vi "故障分解.vi"(3 "名称":string[](array[string]), 5 "故障输入口":string[](array[string])) -> (0 "故障等级":dbl, 1 "输出数组":string[][](array[string]), 2 "故障显示":string[][](array[string]))   [LabVIEW 2013]
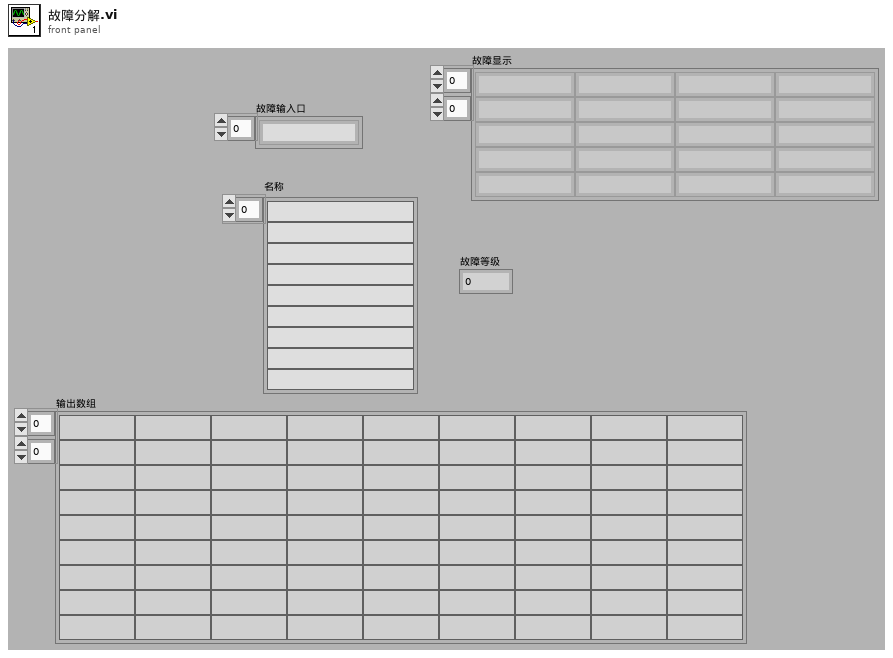
[diagram p1: front panel]
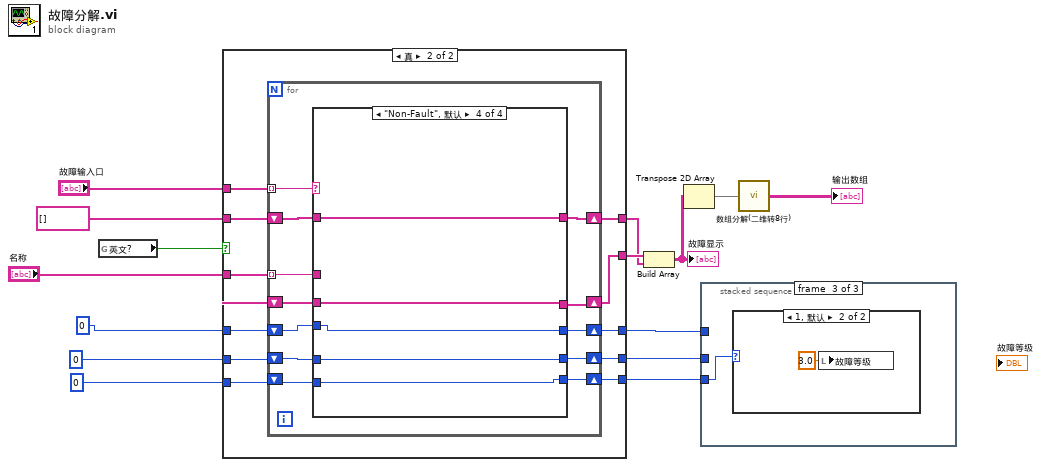
[diagram p0: block diagram]
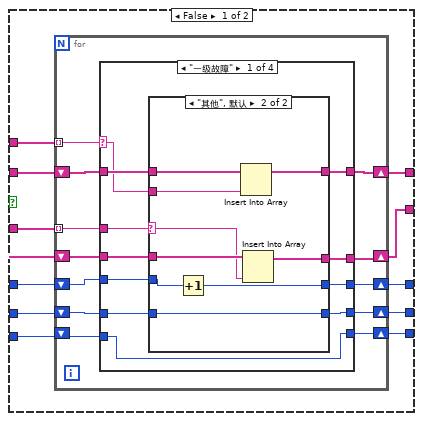
[diagram p2: hidden frame]
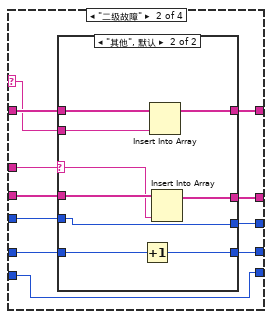
[diagram p4: hidden frame]
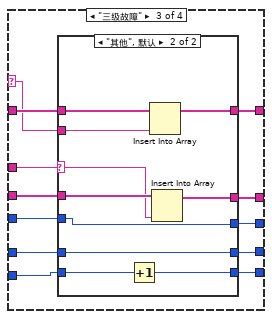
[diagram p6: hidden frame]
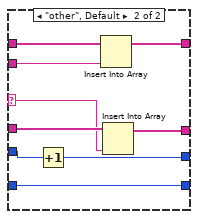
[diagram p10: hidden frame]
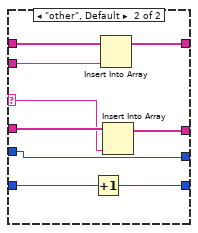
[diagram p12: hidden frame]
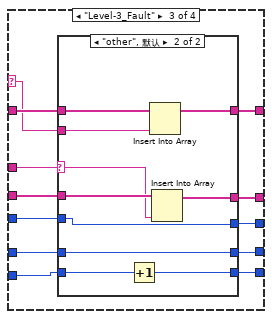
[diagram p13: hidden frame]
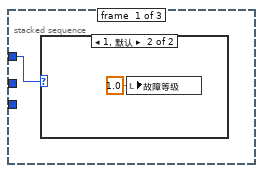
[diagram p15: hidden frame]
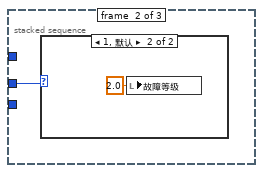
[diagram p17: hidden frame]
diagram:
  n1 = global read "中英文全局-8.6.vi" "英文?"() -> (w1:bool)
  n2 = case shown="真" w1 {
    tunnel: "名称" -> [w26 w129]
    tunnel: string[] [] -> [w25 w128]
    tunnel: 0 ("数值") -> [w24 w127]
    tunnel: 0 ("数值") -> [w23 w126]
    tunnel: 0 ("数值") -> [w22 w125]
    tunnel: [w21 w124] -> w9
    tunnel: [w20 w123] -> w8
    tunnel: [w19 w122] -> w7
    tunnel: [w18 w121] -> w6
    tunnel: [w17 w120] -> w5
    tunnel: "故障输入口" -> [w16 w119]
    frame False {
      n3 = for {
        tunnel: w16 -> [w38] mode=indexing
        tunnel: w26 -> [w35] mode=indexing
        shift-right: [w37] -> w20
        shift-left: w25 -> [w36]
        shift-right: [w33] -> w21
        shift-left: w25 -> [w34]
        shift-right: [w31] -> w19
        shift-left: w24 -> [w32]
        shift-right: [w29] -> w18
        shift-left: w23 -> [w30]
        shift-right: [w27] -> w17
        shift-left: w22 -> [w28]
        n4 = case shown="\"一级故障\"" w38 {
          selector: w38 -> [w47 w71 w96 _]
          tunnel: [w49 w73 w98 w118] -> w37
          tunnel: w36 -> [w48 w72 w97 w118]
          tunnel: w35 -> [w46 w70 w95 _]
          tunnel: w34 -> [w45 w69 w94 w117]
          tunnel: [w44 w68 w93 w117] -> w33
          tunnel: w32 -> [w43 w67 w92 w116]
          tunnel: [w42 w66 w91 w116] -> w31
          tunnel: w30 -> [w40 w65 w90 w115]
          tunnel: [w41 w64 w89 w115] -> w29
          tunnel: w28 -> [w39 w63 w88 w114]
          tunnel: [w39 w63 w87 w114] -> w27
          frame "一级故障" {
            n5 = case shown="\"其他\", 默认" w46 {
              selector: w46 -> [_ w57]
              tunnel: [w53 w62] -> w49
              tunnel: w48 -> [w53 w61]
              tunnel: w47 -> [_ w60]
              tunnel: w45 -> [w52 w59]
              tunnel: [w52 w58] -> w44
              tunnel: [w51 w55] -> w42
              tunnel: w43 -> [w51 w56]
              tunnel: [w50 w54] -> w41
              tunnel: w40 -> [w50 w54]
              frame "保留" {
              }
              frame "其他", Default {
                n6 = Increment(x=w56) -> (x+1=w55:i32)
                n7 = Insert Into Array(array=w61, new element=w60) -> (w62:string[])  [unwired: 1 in]
                n8 = Insert Into Array(array=w59, new element=w57) -> (w58:string[])  [unwired: 1 in]
              }
            }
          }
          frame "二级故障" {
            n9 = case shown="\"其他\", 默认" w70 {
              selector: w70 -> [_ w81]
              tunnel: [w77 w86] -> w73
              tunnel: w72 -> [w77 w85]
              tunnel: w71 -> [_ w84]
              tunnel: w69 -> [w76 w83]
              tunnel: [w76 w82] -> w68
              tunnel: [w75 w80] -> w66
              tunnel: w67 -> [w75 w80]
              tunnel: w65 -> [w74 w79]
              tunnel: [w74 w78] -> w64
              frame "保留" {
              }
              frame "其他", Default {
                n10 = Increment(x=w79) -> (x+1=w78:i32)
                n11 = Insert Into Array(array=w85, new element=w84) -> (w86:string[])  [unwired: 1 in]
                n12 = Insert Into Array(array=w83, new element=w81) -> (w82:string[])  [unwired: 1 in]
              }
            }
          }
          frame "三级故障" {
            n13 = case shown="\"其他\", 默认" w95 {
              selector: w95 -> [_ w108]
              tunnel: [w103 w113] -> w98
              tunnel: w97 -> [w103 w112]
              tunnel: w96 -> [_ w111]
              tunnel: w94 -> [w102 w110]
              tunnel: [w102 w109] -> w93
              tunnel: [w101 w107] -> w91
              tunnel: w92 -> [w101 w107]
              tunnel: w90 -> [w100 w106]
              tunnel: [w100 w106] -> w89
              tunnel: w88 -> [w99 w105]
              tunnel: [w99 w104] -> w87
              frame "保留" {
              }
              frame "其他", Default {
                n14 = Increment(x=w105) -> (x+1=w104:i32)
                n15 = Insert Into Array(array=w112, new element=w111) -> (w113:string[])  [unwired: 1 in]
                n16 = Insert Into Array(array=w110, new element=w108) -> (w109:string[])  [unwired: 1 in]
              }
            }
          }
          frame "无故障", Default {
          }
        }
      }
    }
    frame True {
      n17 = for {
        tunnel: w119 -> [w141] mode=indexing
        tunnel: w129 -> [w138] mode=indexing
        shift-right: [w140] -> w123
        shift-left: w128 -> [w139]
        shift-right: [w136] -> w124
        shift-left: w128 -> [w137]
        shift-right: [w134] -> w122
        shift-left: w127 -> [w135]
        shift-right: [w132] -> w121
        shift-left: w126 -> [w133]
        shift-right: [w130] -> w120
        shift-left: w125 -> [w131]
        n18 = case shown="\"Non-Fault\", 默认" w141 {
          selector: w141 -> [w150 w174 w199 _]
          tunnel: [w152 w176 w201 w221] -> w140
          tunnel: w139 -> [w151 w175 w200 w221]
          tunnel: w138 -> [w149 w173 w198 _]
          tunnel: w137 -> [w148 w172 w197 w220]
          tunnel: [w147 w171 w196 w220] -> w136
          tunnel: w135 -> [w146 w170 w195 w219]
          tunnel: [w145 w169 w194 w219] -> w134
          tunnel: w133 -> [w143 w168 w193 w218]
          tunnel: [w144 w167 w192 w218] -> w132
          tunnel: w131 -> [w142 w166 w191 w217]
          tunnel: [w142 w166 w190 w217] -> w130
          frame "Level-1_Fault" {
            n19 = case shown="\"rsv\"" w149 {
              selector: w149 -> [_ w160]
              tunnel: [w156 w165] -> w152
              tunnel: w151 -> [w156 w164]
              tunnel: w150 -> [_ w163]
              tunnel: w148 -> [w155 w162]
              tunnel: [w155 w161] -> w147
              tunnel: [w154 w158] -> w145
              tunnel: w146 -> [w154 w159]
              tunnel: [w153 w157] -> w144
              tunnel: w143 -> [w153 w157]
              frame "rsv" {
              }
              frame "other", Default {
                n20 = Increment(x=w159) -> (x+1=w158:i32)
                n21 = Insert Into Array(array=w164, new element=w163) -> (w165:string[])  [unwired: 1 in]
                n22 = Insert Into Array(array=w162, new element=w160) -> (w161:string[])  [unwired: 1 in]
              }
            }
          }
          frame "Level-2_Fault" {
            n23 = case shown="\"rsv\"" w173 {
              selector: w173 -> [_ w184]
              tunnel: [w180 w189] -> w176
              tunnel: w175 -> [w180 w188]
              tunnel: w174 -> [_ w187]
              tunnel: w172 -> [w179 w186]
              tunnel: [w179 w185] -> w171
              tunnel: [w178 w183] -> w169
              tunnel: w170 -> [w178 w183]
              tunnel: w168 -> [w177 w182]
              tunnel: [w177 w181] -> w167
              frame "rsv" {
              }
              frame "other", Default {
                n24 = Increment(x=w182) -> (x+1=w181:i32)
                n25 = Insert Into Array(array=w188, new element=w187) -> (w189:string[])  [unwired: 1 in]
                n26 = Insert Into Array(array=w186, new element=w184) -> (w185:string[])  [unwired: 1 in]
              }
            }
          }
          frame "Level-3_Fault" {
            n27 = case shown="\"other\", 默认" w198 {
              selector: w198 -> [_ w211]
              tunnel: [w206 w216] -> w201
              tunnel: w200 -> [w206 w215]
              tunnel: w199 -> [_ w214]
              tunnel: w197 -> [w205 w213]
              tunnel: [w205 w212] -> w196
              tunnel: [w204 w210] -> w194
              tunnel: w195 -> [w204 w210]
              tunnel: w193 -> [w203 w209]
              tunnel: [w203 w209] -> w192
              tunnel: w191 -> [w202 w208]
              tunnel: [w202 w207] -> w190
              frame "rsv" {
              }
              frame "other", Default {
                n28 = Increment(x=w208) -> (x+1=w207:i32)
                n29 = Insert Into Array(array=w215, new element=w214) -> (w216:string[])  [unwired: 1 in]
                n30 = Insert Into Array(array=w213, new element=w211) -> (w212:string[])  [unwired: 1 in]
              }
            }
          }
          frame "Non-Fault", Default {
          }
        }
      }
    }
  }
  n31 = Build Array(w9, w8) -> (w10:string[][])
  "故障显示" <- w10
  n32 = Transpose 2D Array(2D array=w10) -> (transposed array=w3:string[][])
  n33 = stacked-sequence {
    tunnel: w7 -> [w222 _ _]
    tunnel: w6 -> [_ w224 _]
    tunnel: w5 -> [_ _ w226]
    frame #0 {
      n34 = case shown="1, 默认" w222 {
        frame 0 {
        }
        frame 1, Default {
          n35 = local write "故障等级"(1.0 ("故障等级")) -> ()
        }
      }
    }
    frame #1 {
      n36 = case shown="1, 默认" w224 {
        frame 0 {
        }
        frame 1, Default {
          n37 = local write "故障等级"(2.0 ("故障等级")) -> ()
        }
      }
    }
    frame #2 {
      n38 = case shown="1, 默认" w226 {
        frame 0 {
        }
        frame 1, Default {
          n39 = local write "故障等级"(3.0 ("故障等级")) -> ()
        }
      }
    }
  }
  n40 = call "数组分解(二维转8行).vi"("输入数组"=w3) -> ("输出数组"=→"输出数组":string[][])
